vi "RP get info.vi"(5 "Ranges":dbl[](array[numeric])=[20.0, 1.0], 7 "Trigger offset":i32 format="0x%x (%d)", 8 "Error In":errorcluster, 9 "Channel names":string[](array[string])=["CH0", "CH1"], 11 "connection ID":refnum<k5>) -> (0 "Error Out":errorcluster, 2 "Channel info":T1[](array[typedef]) {"waveform start" format="%#_6p"; "waveform period" format="%#_6p"}, 3 "connection ID out":refnum<k5>)   [LabVIEW 2015]
uses:
  RP info.ctl
panel:
  out "Status response 2":u32=1 format="0x%x (%d)"
  out "Status response":u32=1 format="0x%x (%d)"
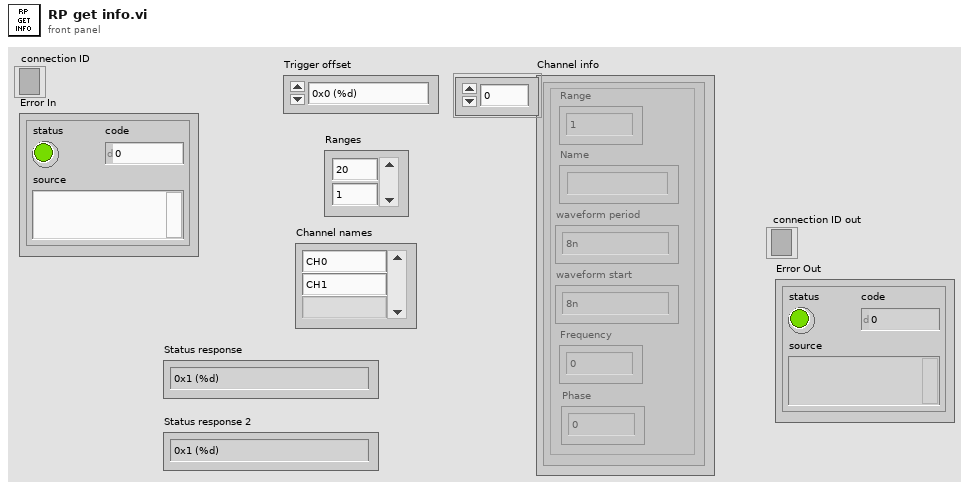
[diagram p1: front panel]
types:
  T1 = typedef "RP info.ctl" = cluster{"Range":dbl, "Name":string, "waveform period":dbl, "waveform start":dbl, "Frequency":u32, "Phase":u32}
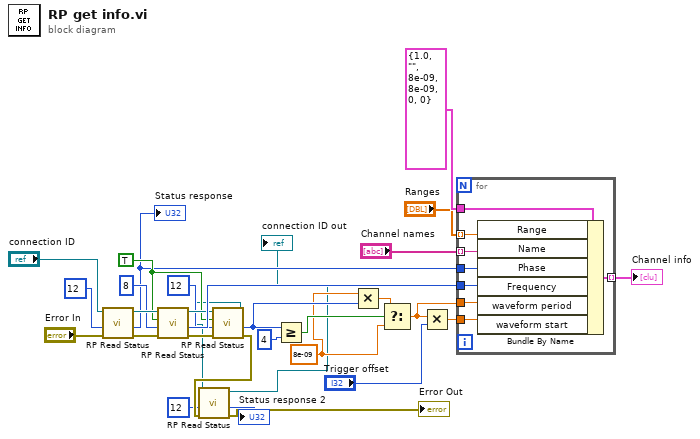
[diagram p0: block diagram]
diagram:
  w11 = 8e-09
  w17 = TRUE ("Read config")
  n1 = call "RP Read Status.vi"("Error In"="Error In", "Status offset"=u64 12, "connection ID"="connection ID") -> ("Error Out"=w21:errorcluster, "Status response"=w7:u32, "connection ID out"=w23:refnum<k5>)  [unwired: 6 in]
  "Status response" <- w7
  n2 = call "RP Read Status.vi"("Error In"=w21, "Status offset"=u64 8, "Read config"=w17, "connection ID"=w23) -> ("Error Out"=w16:errorcluster, "Status response"=w20:u32, "connection ID out"=w19:refnum<k5>)  [unwired: 5 in]
  n3 = call "RP Read Status.vi"("Error In"=w16, "Status offset"=u64 12, "Read config"=w17, "connection ID"=w19) -> ("Error Out"=w5:errorcluster, "Status response"=w14:u32, "connection ID out"=w4:refnum<k5>)  [unwired: 5 in]
  n4 = call "RP Read Status.vi"("Error In"=w5, "Status offset"=u64 12, "connection ID"=w4) -> ("Error Out"=→"Error Out":errorcluster, "Status response"=→"Status response 2":u32, "connection ID out"=→"connection ID out":refnum<k5>)  [unwired: 6 in]
  n5 = Greater Or Equal?(x=w14, y=u32 4) -> (x >= y?=w12:bool)
  n6 = Multiply(x=w11, y=w14) -> (x*y=w13:dbl)
  n7 = Select(t=w13, s=w12, f=w11) -> (s? t:f=w9:dbl)
  n8 = Multiply(x=w9, y="Trigger offset") -> (x*y=w8:dbl)
  n9 = for {
    tunnel: T1 {"Range"=1.0, "Name"="", "waveform period"=8e-09, "waveform start"=8e-09, "Frequency"=0, "Phase"=0} ("RP info") -> [w38]
    tunnel: "Ranges" -> [w37] mode=indexing
    tunnel: "Channel names" -> [w36] mode=indexing
    tunnel: [w35] -> w24 mode=indexing
    tunnel: w7 -> [w34]
    tunnel: w20 -> [w33]
    tunnel: w9 -> [w32]
    tunnel: w8 -> [w31]
    n10 = Bundle By Name(cluster=w38, "Range"=w37, "Name"=w36, "Phase"=w34, "Frequency"=w33, "waveform period"=w32, "waveform start"=w31) -> (w35:T1)
  }
  "Channel info" <- w24
